vi "2025_Version.vi"() -> ()   [LabVIEW 2025]
uses:
  <vilib>/ErrorRing/Error Ring.xnode
panel:
  in  "Instructions":bool
  out "Test":string
  out "Index_Display":i32
  out "Score":i32
  in  "Start Button":bool
  in  "Boolean 4":bool
  in  "Boolean 3":bool
  in  "Boolean 2":bool
  in  "Boolean":bool
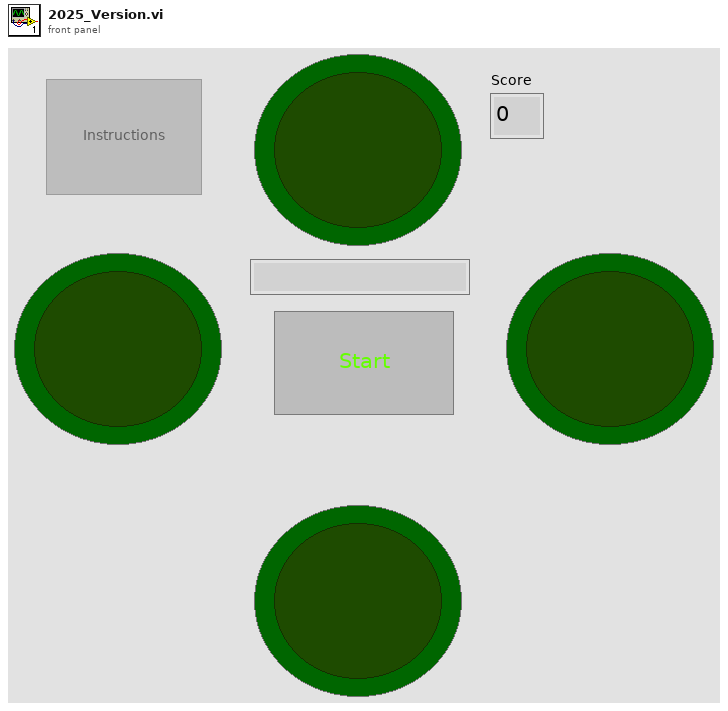
[diagram p1: front panel]
types:
  T1 = enum8{"Enabled", "Disabled", "Disabled and Grayed Out"}
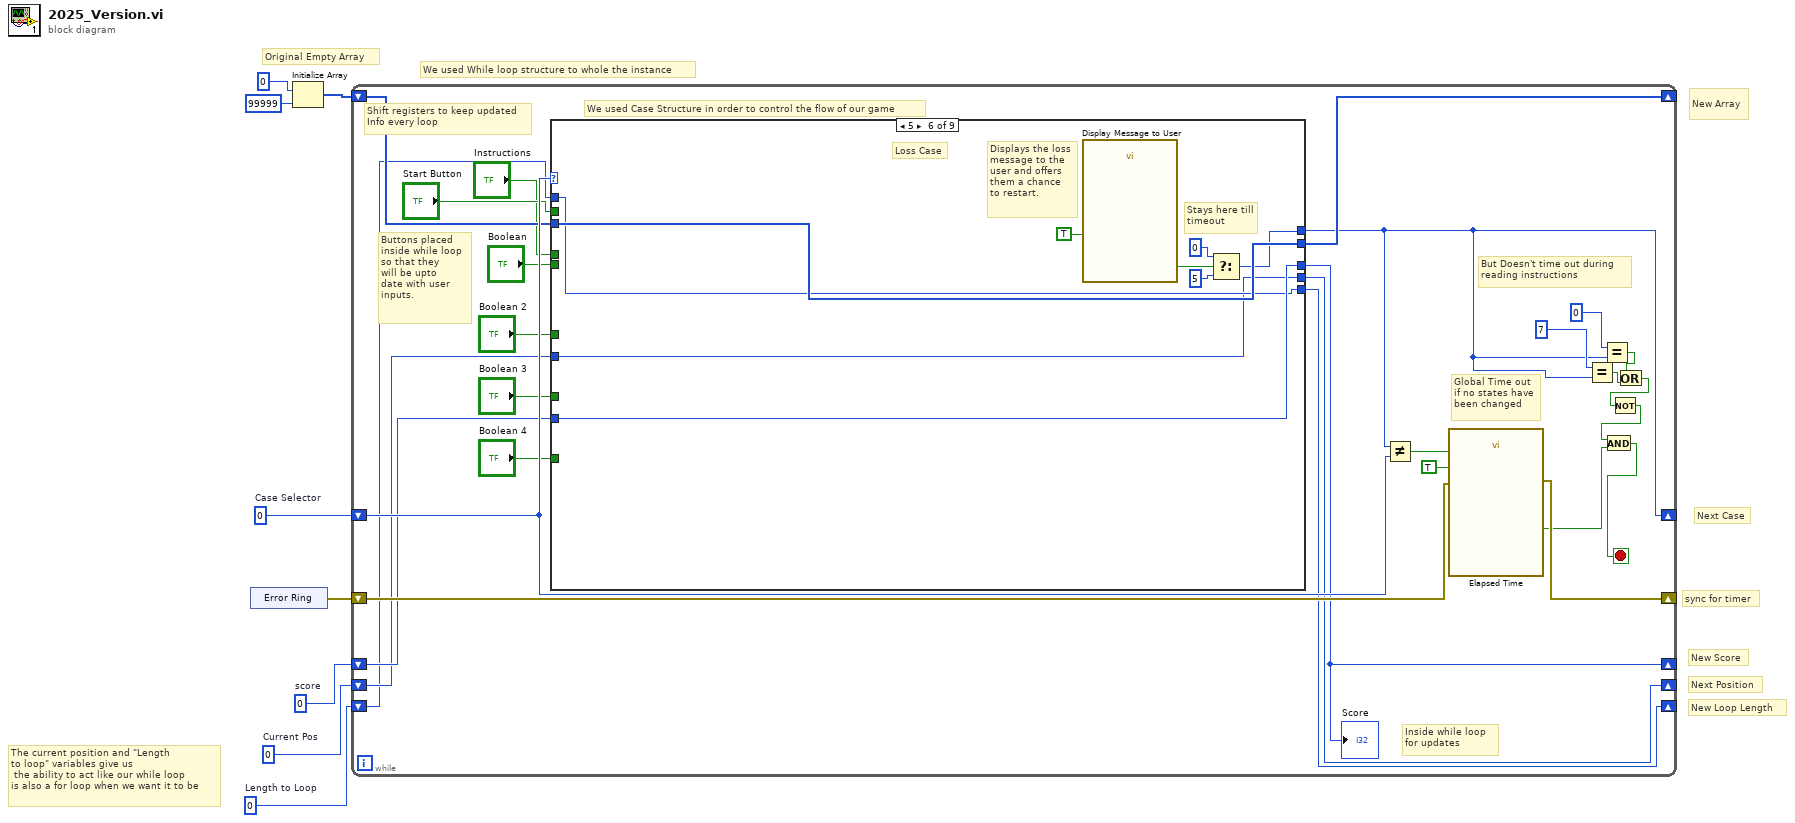
[diagram p0: block diagram]
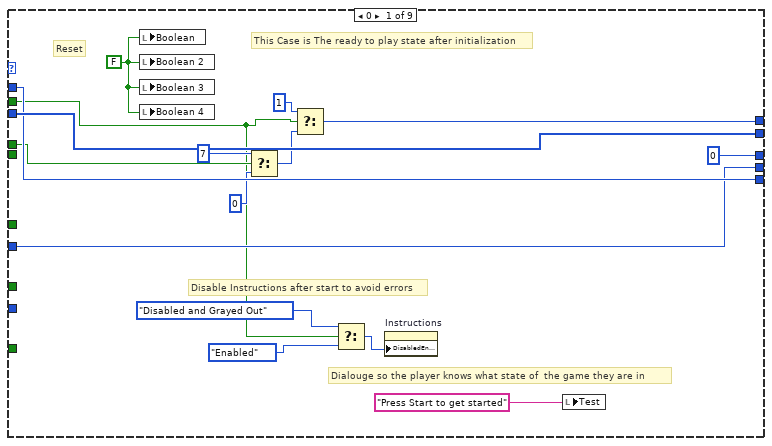
[diagram p2: hidden frame]
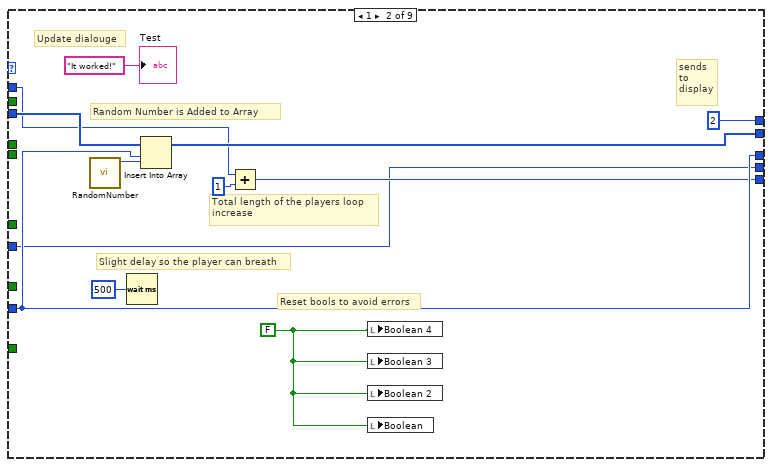
[diagram p3: hidden frame]
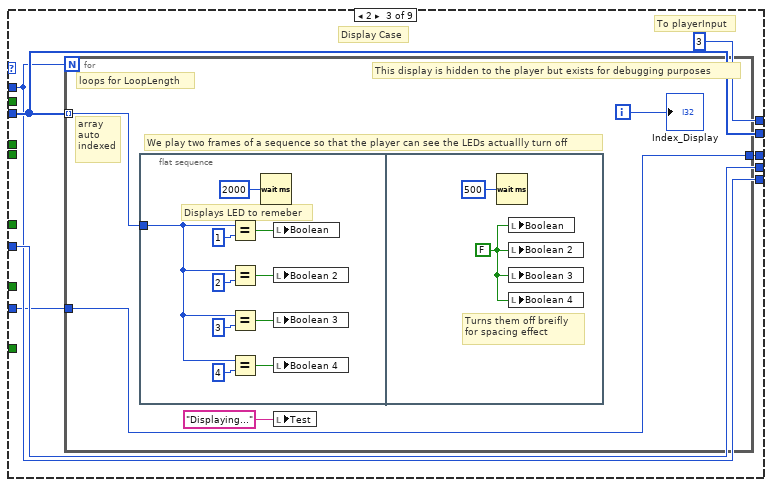
[diagram p4: hidden frame]
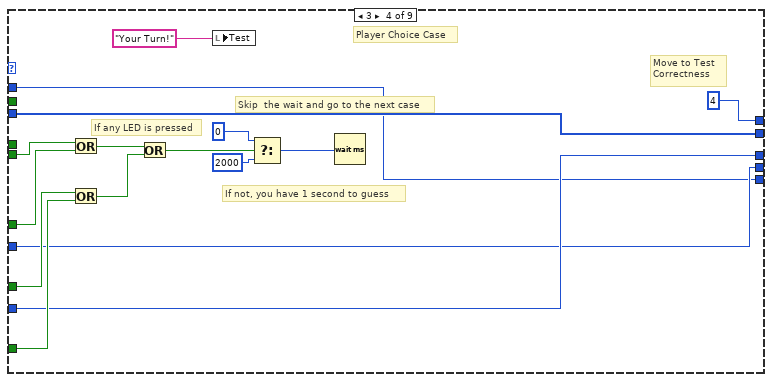
[diagram p5: hidden frame]
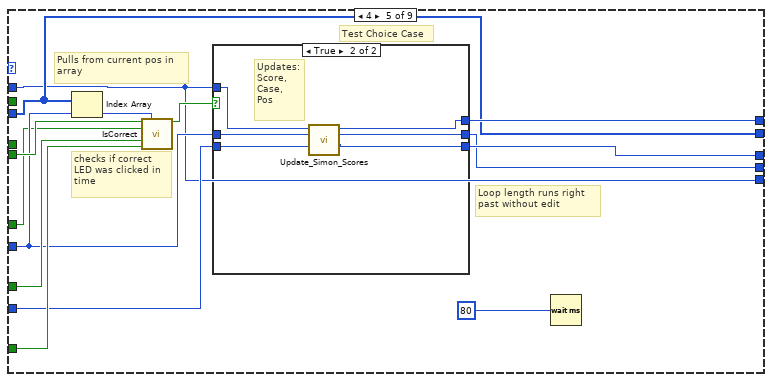
[diagram p6: hidden frame]
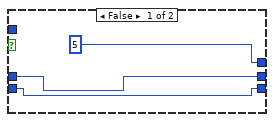
[diagram p7: hidden frame]
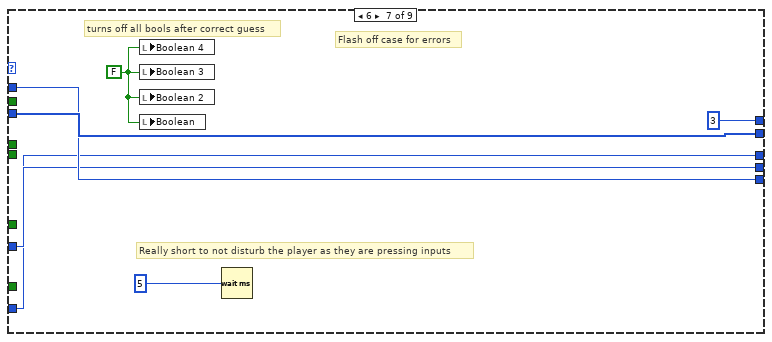
[diagram p8: hidden frame]
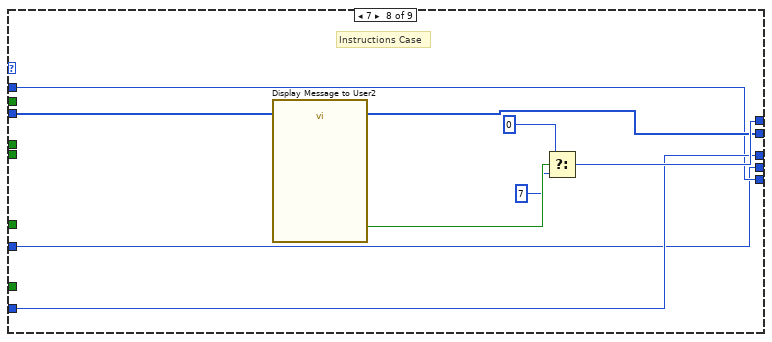
[diagram p9: hidden frame]
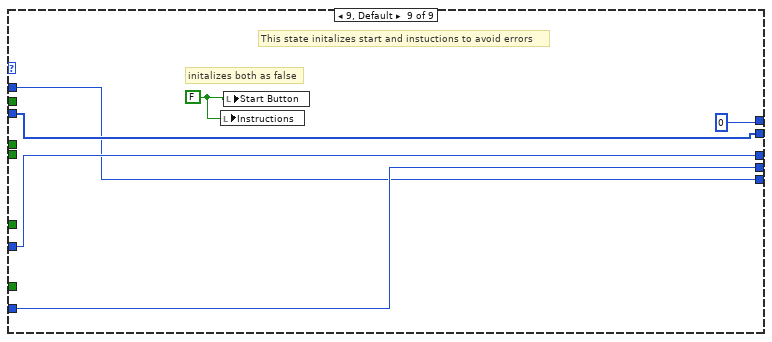
[diagram p10: hidden frame]
diagram:
  w2 = 0  # Length to Loop
  w3 = 0  # Current Pos
  w7 = 0  # score
  w8 = 0  # Case Selector
  # "We used While loop structure to whole the instance"
  # "sync for timer"
  # "New Loop Length"
  # "Next Position"
  # "New Score"
  # "Next Case"
  # "New Array"
  # "The current position and \"Length \nto loop\" variables give us\n the ability to act like our while loop\nis also a for loop when we want it to be"
  # "Original Empty Array"
  n1 = xnode "Error Ring"() -> ("error out"=w1:errorcluster)
  n2 = Initialize Array(0 ("element"), 99999 ("dimension size")) -> (w4:i32[])
  n3 = while {
    shift-right: [w34] -> _
    shift-left: w1 -> [w33]
    shift-right: [w9] -> _
    shift-left: w8 -> [w32]
    shift-right: [w28] -> _
    shift-left: w7 -> [w30]
    shift-right: [w29] -> _
    shift-left: w4 -> [w31]
    shift-right: [w25] -> _
    shift-left: w2 -> [w26]
    shift-right: [w24] -> _
    shift-left: w3 -> [w27]
    stop <- w15 stop-if-true
    # "We used Case Structure in order to control the flow of our game"
    # "But Doesn't time out during\nreading instructions"
    # "Global Time out\nif no states have\nbeen changed"
    # "Inside while loop \nfor updates"
    # "Buttons placed\ninside while loop\nso that they \nwill be upto\ndate with user\ninputs."
    # "Shift registers to keep updated \nInfo every loop"
    n4 = case shown="5" w32 {
      tunnel: "Start Button" -> [w40 _ _ _ _ _ _ _ _]
      tunnel: [w51 2 ("f") 3 ("f") 4 ("f") w110 w129 3 ("f") w146 0 ("f")] -> w9
      tunnel: w31 -> [w49 w63 w70 w91 w108 w134 w140 w144 w154]
      tunnel: w30 -> [_ w59 w65 w90 w112 w128 w137 w145 w152]
      tunnel: [w49 w62 w70 w91 w108 w134 w140 w144 w154] -> w29
      tunnel: [0 ("score") w59 w66 w90 w111 w128 w137 w145 w153] -> w28
      tunnel: "Boolean" -> [_ _ _ w100 w116 _ _ _ _]
      tunnel: "Boolean 2" -> [_ _ _ w99 w103 _ _ _ _]
      tunnel: "Boolean 3" -> [_ _ _ w98 w115 _ _ _ _]
      tunnel: "Boolean 4" -> [_ _ _ w97 w114 _ _ _ _]
      tunnel: w27 -> [w47 w55 w69 w89 w107 w126 w138 w142 w153]
      tunnel: w26 -> [w48 w58 w67 w88 w105 w127 w139 w143 w151]
      tunnel: [w48 w56 w67 w88 w105 w127 w139 w143 w151] -> w25
      tunnel: [w47 w55 w69 w89 w106 w126 w138 w142 w152] -> w24
      tunnel: "Instructions" -> [w44 _ _ _ _ _ _ _ _]
      frame 0 {
        w46 = FALSE ("Boolean")
        # "Disable Instructions after start to avoid errors"
        # "Dialouge so the player knows what state of  the game they are in"
        # "This Case is The ready to play state after initialization"
        # "Reset"
        n5 = local write "Boolean"(w46) -> ()
        n6 = local write "Boolean 2"(w46) -> ()
        n7 = local write "Boolean 3"(w46) -> ()
        n8 = local write "Boolean 4"(w46) -> ()
        n9 = Select(t=7, s=w44, f=0 ("t")) -> (s? t:f=w42:i32)
        n10 = Select(t=1, s=w40, f=w42) -> (s? t:f=w51:i32)
        n11 = Select(t=T1."Disabled and Grayed Out" ("Disabled"), s=w40, f=T1."Enabled" ("Disabled")) -> (s? t:f=w37:T1)
        n12 = property on="Instructions" class="Bool (strict)"("DisabledEnum"=w37) -> ()  [unwired: 2 in, 2 out]
        n13 = local write "Test"("Press Start to get started" ("Test")) -> ()
      }
      frame 1 {
        w53 = FALSE ("Boolean 4")
        # "sends\nto\ndisplay"
        # "Reset bools to avoid errors"
        # "Slight delay so the player can breath"
        # "Total length of the players loop\nincrease"
        # "Random Number is Added to Array"
        # "Update dialouge"
        n14 = call "RandomNumber.vi"() -> ("Numeric"=w61:i32)  [unwired: 11 in]
        n15 = Wait (ms)(milliseconds to wait=u32 500) -> ()  [unwired: 1 out]
        n16 = Insert Into Array(array=w63, index=w59, new element=w61) -> (w62:i32[])
        n17 = Add(x=w58, y=1) -> (x+y=w56:i32)
        n18 = local write "Boolean 4"(w53) -> ()
        n19 = local write "Boolean 3"(w53) -> ()
        n20 = local write "Boolean 2"(w53) -> ()
        n21 = local write "Boolean"(w53) -> ()
        "Test" <- "It worked!"
      }
      frame 2 {
        # "Display Case"
        # "To playerInput"
        n22 = for {
          N: w67 -> [_]
          tunnel: w70 -> [w73] mode=indexing
          tunnel: w65 -> [w72]
          tunnel: [w72] -> w66
          i -> [w74]
          # "array\nauto\nindexed"
          # "loops for LoopLength"
          # "We play two frames of a sequence so that the player can see the LEDs actuallly turn off"
          # "This display is hidden to the player but exists for debugging purposes"
          n23 = flat-sequence {
            tunnel: w73 -> [w78]
            frame #0 {
              # "Displays LED to remeber"
              n24 = Equal?(x=w78, y=1) -> (x = y?=w84:bool)
              n25 = Equal?(x=w78, y=2) -> (x = y?=w81:bool)
              n26 = Equal?(x=w78, y=3) -> (x = y?=w82:bool)
              n27 = Equal?(x=w78, y=4) -> (x = y?=w83:bool)
              n28 = Wait (ms)(milliseconds to wait=u32 2000) -> ()  [unwired: 1 out]
              n29 = local write "Boolean"(w84) -> ()
              n30 = local write "Boolean 2"(w81) -> ()
              n31 = local write "Boolean 3"(w82) -> ()
              n32 = local write "Boolean 4"(w83) -> ()
            }
            frame #1 {
              w86 = FALSE ("Boolean 4")
              # "Turns them off breifly \nfor spacing effect"
              n33 = Wait (ms)(milliseconds to wait=u32 500 ("x")) -> ()  [unwired: 1 out]
              n34 = local write "Boolean"(w86) -> ()
              n35 = local write "Boolean 2"(w86) -> ()
              n36 = local write "Boolean 3"(w86) -> ()
              n37 = local write "Boolean 4"(w86) -> ()
            }
          }
          n38 = local write "Test"("Displaying..." ("Test")) -> ()
          "Index_Display" <- w74
        }
      }
      frame 3 {
        # "Move to Test \nCorrectness"
        # "Player Choice Case"
        # "If not, you have 1 second to guess"
        # "Skip  the wait and go to the next case"
        # "If any LED is pressed"
        n39 = Or(x=w100, y=w99) -> (x .or. y?=w102:bool)
        n40 = Or(x=w98, y=w97) -> (x .or. y?=w101:bool)
        n41 = Or(x=w102, y=w101) -> (x .or. y?=w96:bool)
        n42 = local write "Test"("Your Turn!" ("Test")) -> ()
        n43 = Select(t=u32 0 ("milliseconds to wait"), s=w96, f=u32 2000 ("milliseconds to wait")) -> (s? t:f=w93:u32)
        n44 = Wait (ms)(milliseconds to wait=w93) -> ()  [unwired: 1 out]
      }
      frame 4 {
        # "Test Choice Case"
        # "Pulls from current pos in\narray"
        # "Loop length runs right \npast without edit"
        # "checks if correct\nLED was clicked in\ntime"
        n45 = Index Array(array=w108, index=w107) -> (element=w113:i32)
        n46 = call "IsCorrect.vi"("Boolean"=w116, "InValue"=w113, "Boolean 2"=w103, "Boolean 3"=w115, "Boolean 4"=w114) -> ("IsCorrect"=w109:bool)  [unwired: 10 in]
        n47 = case shown="True" w109 {
          tunnel: [5 ("f") w121] -> w110
          tunnel: w112 -> [w118 w123]
          tunnel: [w118 w122] -> w111
          tunnel: w107 -> [w117 w124]
          tunnel: [w117 w120] -> w106
          tunnel: w105 -> [_ w125]
          frame False {
          }
          frame True {
            # "Updates:\nScore,\nCase,\nPos"
            n48 = call "Update_Simon_Scores.vi"("Score"=w123, "Position"=w124, "LoopLength"=w125) -> ("New Score"=w122:i32, "Next Pos"=w120:i32, "Case Selector"=w121:i32)  [unwired: 6 in]
          }
        }
        n49 = Wait (ms)(milliseconds to wait=u32 80) -> ()  [unwired: 1 out]
      }
      frame 5 {
        # "Loss Case"
        # "Stays here till\ntimeout"
        # "Displays the loss\nmessage to the \nuser and offers\nthem a chance \nto restart."
        n50 = call "Display Message to User"("Enable"=TRUE) -> ("OK"=w132:bool)  [unwired: 9 in, 1 out]
        n51 = Select(t=0, s=w132, f=5) -> (s? t:f=w129:i32)
      }
      frame 6 {
        w136 = FALSE ("Boolean 4")
        # "turns off all bools after correct guess"
        # "Really short to not disturb the player as they are pressing inputs"
        # "Flash off case for errors"
        n52 = local write "Boolean 4"(w136) -> ()
        n53 = local write "Boolean 3"(w136) -> ()
        n54 = local write "Boolean 2"(w136) -> ()
        n55 = local write "Boolean"(w136) -> ()
        n56 = Wait (ms)(milliseconds to wait=u32 5) -> ()  [unwired: 1 out]
      }
      frame 7 {
        # "Instructions Case"
        n57 = call "Display Message to User2"() -> ("OK"=w149:bool)  [unwired: 10 in, 1 out]
        n58 = Select(t=0 ("f"), s=w149, f=7) -> (s? t:f=w146:i32)
      }
      frame 9, Default {
        w150 = FALSE ("Start Button")
        # "initalizes both as false"
        # "This state initalizes start and instuctions to avoid errors"
        n59 = local write "Instructions"(w150) -> ()
        n60 = local write "Start Button"(w150) -> ()
      }
    }
    "Score" <- w28
    n61 = Not Equal?(x=w9, y=w32) -> (x != y?=w35:bool)
    n62 = call "Elapsed Time"("Reset"=w35, "Auto Reset"=TRUE, "error in (no error)"=w33) -> ("Time has Elapsed"=w16:bool, "error out"=w34:errorcluster)  [unwired: 9 in, 6 out]
    n63 = Equal?(x=7 ("t"), y=w9) -> (x = y?=w13:bool)
    n64 = Equal?(x=0 ("t"), y=w9) -> (x = y?=w12:bool)
    n65 = Or(x=w12, y=w13) -> (x .or. y?=w11:bool)
    n66 = Not(x=w11) -> (.not. x?=w10:bool)
    n67 = And(x=w10, y=w16) -> (x .and. y?=w15:bool)
  }
